vi "setSpectTempSetpoint.vi"(8 "error in (no error)":errorcluster, 9 "command_setSpectTempSetpoint":T1, 10 "model in":refnum<class "IModel.lvclass">, 11 "DefaultState in":refnum<class "DefaultState.lvclass">) -> (0 "error out":errorcluster, 2 "model out":refnum<class "IModel.lvclass">, 3 "DefaultState out":refnum<class "DefaultState.lvclass">)   [LabVIEW 2016, in "States.lvlib" / "DefaultState.lvclass"]
uses:
  DefaultState.lvclass
  IModel/IModel.lvclass
  ts_sallv_sedspectrometer/DataTypes/command_setSpectTempSetpoint.ctl
  Typedefs/CommandValue.ctl
  Typedefs/SEDSpectrometerTypedefs.lvlib
  ts_sallv_sedspectrometer/SALLV_sedSpectrometer.lvlib
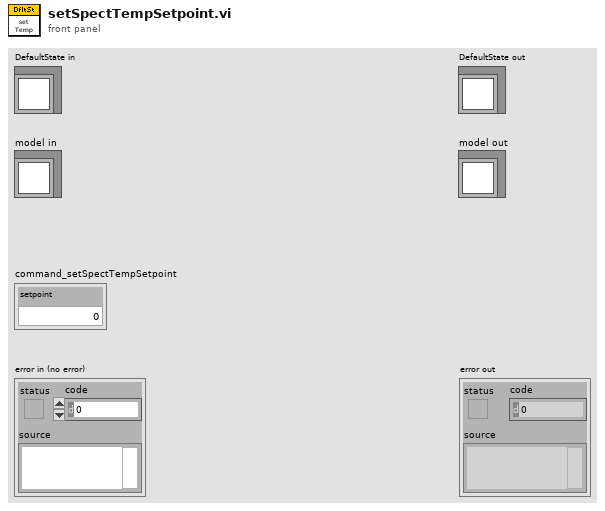
[diagram p1: front panel]
types:
  T1 = typedef "SALLV_sedSpectrometer.lvlib/command_setSpectTempSetpoint.ctl" = cluster{"setpoint":sgl}
  T2 = typedef "SEDSpectrometerTypedefs.lvlib/CommandValue.ctl" = enum16{"clearError", "disable", "enable", "exit", "GoToStandby", "OnHeartbeat", "OnIncomingMessagingError", "OnInterrupt", "start", "captureSpectImage", "setSpectTempSetpoint", "stopImageCapture"}
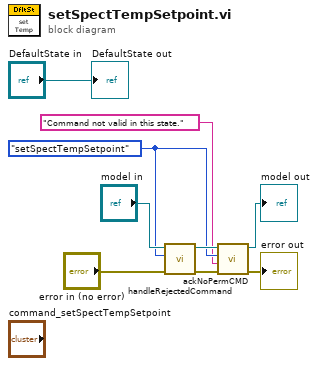
[diagram p0: block diagram]
diagram:
  w2 = CommandValue."setSpectTempSetpoint" ("CommandValue")
  n1 = call-dynamic "handleRejectedCommand.vi"("error in (no error)"="error in (no error)", "CommandValue"=w2, "IModel in"="model in") -> ("error out"=w4:errorcluster, "IModel out"=w6:refnum<class "IModel.lvclass">)  [unwired: 7 in]
  n2 = call-dynamic "ackNoPermCMD.vi"("error in (no error)"=w4, "rejectedReason"="Command not valid in this state.", "CommandValue"=w2, "IModel in"=w6) -> ("error out"=→"error out":errorcluster, "IModel out"=→"model out":refnum<class "IModel.lvclass">)  [unwired: 6 in]
  "DefaultState out" <- "DefaultState in"
